vi "Parameters.vi"() -> ()   [LabVIEW 2013]
uses:
  Parameters/GetSystemParameterInteger.vi
  Parameters/GetAxisParameterDouble.vi
  Parameters/GetAxisParameterString.vi
  Parameters/GetTaskParameterDouble.vi
  Parameters/SetSystemParameterInteger.vi
  Parameters/SetAxisParameterDouble.vi
  Parameters/SetAxisParameterString.vi
  Parameters/SetTaskParameterDouble.vi
panel:
  out "DefaultSCurve":dbl
  out "Error Status":bool
  in  "Send":bool caption="Save"
  out "error out":errorcluster
  in  "Parameter File":path=path "C:/ensemble.prme" caption="File Name and Path"
  out "UnitsName":string
  out "CountsPerUnit":dbl
  out "SerialPort0BaudRate":i32
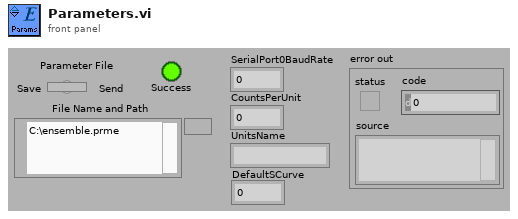
[diagram p1: front panel]
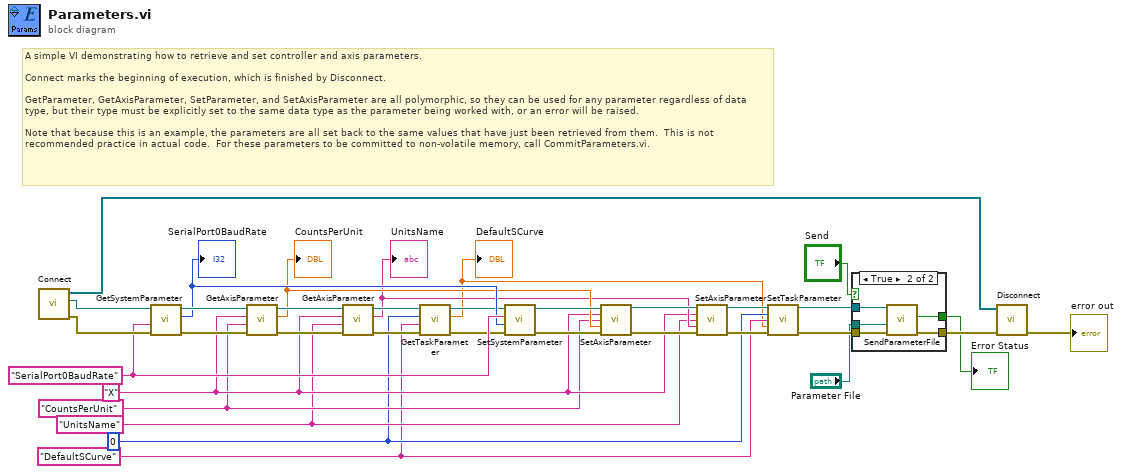
[diagram p0: block diagram]
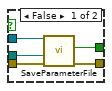
[diagram p2: hidden frame]
diagram:
  w2 = "DefaultSCurve" ("paramName")
  w3 = 0 ("Task Number")
  w18 = "X" ("axisName")
  w16 = "UnitsName" ("paramName")
  w17 = "CountsPerUnit" ("paramName")
  w22 = "SerialPort0BaudRate" ("paramName")
  # "A simple VI demonstrating how to retrieve and set controller and axis parameters.\n\nConnect marks the beginning of execution, which is finished by Disconnect.\n\nGetParameter, GetAxisParameter, SetParameter, and SetAxisParameter are all polymorphic, so they can be used for any parameter regardless of data type, but their type must be explicitly set to the same data type as the parameter being worked with, or an error will be raised.\n\nNote that because this is an example, the parameters are all set back to the same values that have just been retrieved from them.  This is not recommended practice in actual code.  For these parameters to be committed to non-volatile memory, call CommitParameters.vi."
  n1 = call "Connect.vi"() -> ("error out"=w32:errorcluster, "controller"=w33:refnum<k24>, "controllers"=w15:refnum<k24>[])  [unwired: 9 in]
  n2 = call-poly "GetSystemParameter.vi"("error in (no error)"=w32, "Parameter Name"=w22, "controller in"=w33) -> ("error out"=w30:errorcluster, "value"=w21:i32, "controller out"=w31:refnum<k24>)  [unwired: 6 in]
  "SerialPort0BaudRate" <- w21
  n3 = call-poly "GetAxisParameter.vi"("error in (no error)"=w30, "Parameter Name"=w17, "axis name"=w18, "controller in"=w31) -> ("error out"=w28:errorcluster, "value"=w20:dbl, "controller out"=w29:refnum<k24>)  [unwired: 5 in]
  "CountsPerUnit" <- w20
  n4 = call-poly "GetAxisParameter.vi"("error in (no error)"=w28, "Parameter Name"=w16, "axis name"=w18, "controller in"=w29) -> ("error out"=w6:errorcluster, "value"=w19:string, "controller out"=w27:refnum<k24>)  [unwired: 5 in]
  "UnitsName" <- w19
  n5 = call-poly "GetTaskParameter.vi"("error in (no error)"=w6, "Parameter Name"=w2, "task id"=w3, "controller in"=w27) -> ("error out"=w5:errorcluster, "value"=w1:dbl, "controller out"=w7:refnum<k24>)  [unwired: 5 in]
  "DefaultSCurve" <- w1
  n6 = call-poly "SetSystemParameter.vi"("error in (no error)"=w5, "value"=w21, "Parameter Name"=w22, "controller in"=w7) -> ("error out"=w23:errorcluster, "controller out"=w26:refnum<k24>)  [unwired: 4 in]
  n7 = call-poly "SetAxisParameter.vi"("Controller In"=w26, "axisName"=w18, "Parameter Name"=w17, "value"=w20, "error in (no error)"=w23) -> ("Controller Out"=w25:refnum<k24>, "error out"=w24:errorcluster)  [unwired: 9 in]
  n8 = call-poly "SetAxisParameter.vi"("Controller In"=w25, "axisName"=w18, "Parameter Name"=w16, "value"=w19, "error in (no error)"=w24) -> ("Controller Out"=w12:refnum<k24>, "error out"=w14:errorcluster)  [unwired: 9 in]
  n9 = call-poly "SetTaskParameter.vi"("Controller In"=w12, "task id"=w3, "Parameter Name"=w2, "value"=w1) -> ("Controller Out"=w4:refnum<k24>)  [unwired: 10 in, 1 out]
  n10 = case shown="True" "Send" {
    tunnel: w14 -> [w38 w43]
    tunnel: [w37 w42] -> w13
    tunnel: w4 -> [w35 w41]
    tunnel: "Parameter File" -> [w36 w40]
    tunnel: [w34 w39] -> w8
    frame False {
      n11 = call "SaveParameterFile.vi"("error in (no error)"=w38, "Parameter File path and name"=w36, "controller in"=w35) -> ("error out"=w37:errorcluster, "Error Status"=w34:bool)  [unwired: 6 in, 1 out]
    }
    frame True {
      n12 = call "SendParameterFile.vi"("error in (no error)"=w43, "Parameter File path and name"=w40, "controller in"=w41) -> ("error out"=w42:errorcluster, "Error Status"=w39:bool)  [unwired: 6 in, 1 out]
    }
  }
  "Error Status" <- w8
  n13 = call "Disconnect.vi"("error in (no error)"=w13, "controllers"=w15) -> ("error out"=→"error out":errorcluster)  [unwired: 9 in]
